vi "Draw Mono8 to Picture.vi"(7 "Top Left Point (0,0)":T1, 8 "error in (no error)":errorcluster, 11 "Buffer in":refnum<class "Buffer.lvclass">) -> (0 "error out":errorcluster, 2 "Picture":picture, 3 "Buffer":refnum<class "Buffer.lvclass">)   [LabVIEW 2020, in "Buffer.lvclass"]
doc: "Read the buffer data assuming it is in the Mono 8 pixel format and draw it directly to a LabVIEW Picture."
uses:
  Buffer.lvclass
  Picture Top Left Point Offset.ctl
  Pixel Formats.ctl
  Buffer.lvclass/Buffer.ctl
  <vilib>/Utility/error.llb/Error Cluster From Error Code.vi
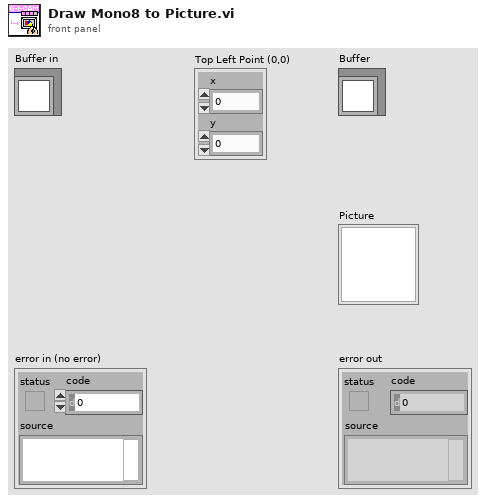
[diagram p1: front panel]
types:
  T1 = typedef "Buffer.lvclass/Picture Top Left Point Offset.ctl" = cluster{"x":i16, "y":i16}
  T2 = typedef "Buffer.lvclass/Pixel Formats.ctl" = enum16{"mono8", "mono10", "mono10p", "mono12", "mono12p", "mono14", "mono14p", "mono16", "RGB8", "BGR8"}
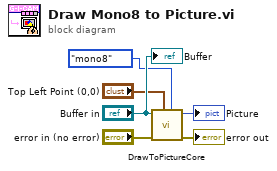
[diagram p0: block diagram]
diagram:
  n1 = call "DrawToPictureCore.vi"("Pixel Formats"=Pixel_Formats."mono8", "Top Left Point"="Top Left Point (0,0)", "error in (no error)"="error in (no error)", "Buffer In"="Buffer in") -> ("error out"=→"error out":errorcluster, "Picture"=→"Picture":picture)  [unwired: 6 in]
  "Buffer" <- "Buffer in"
